vi "SetEntryPatternCode.vi"(1 "Pattern Code Options":u16(ring) items=["Value", "Default", "Minimum", "Maximum"], 3 "error in (no error)":errorcluster, 4 "Pattern Code":u8=1 min=1, 5 "Element":i16=1 min=1, 6 "VISA resource name":refnum<visa-resource-name>) -> (0 "error out":errorcluster, 2 "VISA resource name out":refnum<visa-resource-name>)   [LabVIEW 2020, in "Active Technologies AWG3000.lvlib"]
uses:
  Active Technologies AWG3000.lvlib
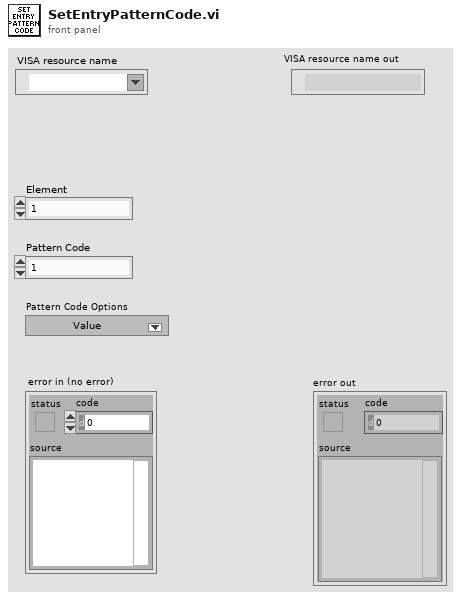
[diagram p1: front panel]
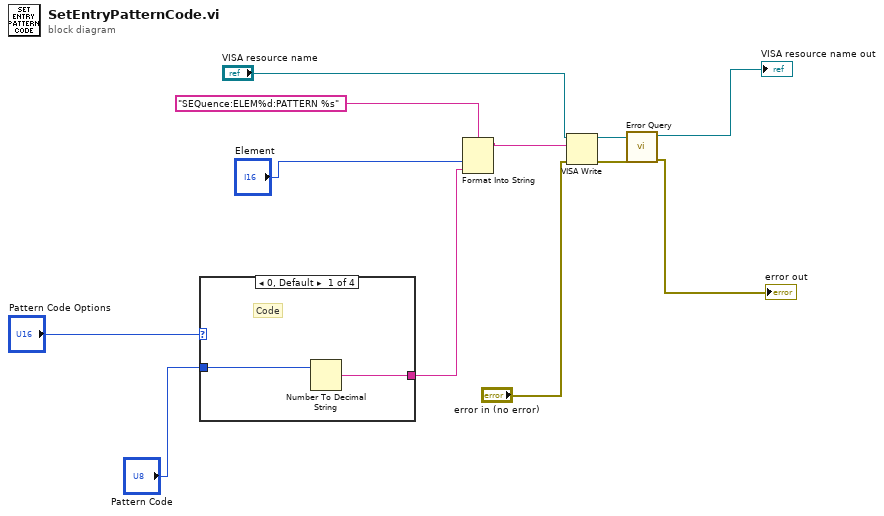
[diagram p0: block diagram]
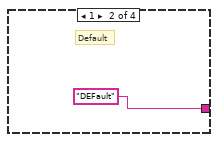
[diagram p2: hidden frame]
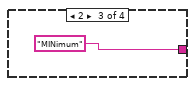
[diagram p3: hidden frame]
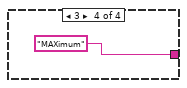
[diagram p4: hidden frame]
diagram:
  n1 = case shown="0, Default" "Pattern Code Options" {
    tunnel: [w14 "DEFault" ("write buffer") "MINimum" ("write buffer") "MAXimum" ("write buffer")] -> w3
    tunnel: "Pattern Code" -> [w13 _ _ _]
    frame 0, Default {
      # "Code"
      n2 = Number To Decimal String(number=w13) -> (decimal integer string=w14:string)  [unwired: 1 in]
    }
    frame 1 {
      # "Default"
    }
    frame 2 {
    }
    frame 3 {
    }
  }
  n3 = Format Into String(format string="SEQuence:ELEM%d:PATTERN %s" ("write buffer"), "Element", w3) -> (resulting string=w4:string)  [unwired: 2 in, 1 out]
  n4 = VISA Write(VISA resource name="VISA resource name", write buffer=w4, error in (no error)="error in (no error)") -> (VISA resource name out=w9:refnum<visa-resource-name>, error out=w8:errorcluster)  [unwired: 1 out]
  n5 = call "Error Query.vi"("error in (no error)"=w8, "VISA resource name"=w9) -> ("error out"=→"error out":errorcluster, "VISA resource name out"=→"VISA resource name out":refnum<visa-resource-name>)  [unwired: 6 in, 2 out]
